vi "AlliGator Image Profile Menu Check Marks.vi"(8 "Error In":errorcluster, 11 "Menu in":refnum<k9>) -> (0 "Error Out":errorcluster)   [LabVIEW 2021, in "AlliGator Image Profile Window.lvlib"]
doc: "Handles checked items in Profile Window menu."
uses:
  AlliGator Image Profile Window.lvlib
  Globals, Variables, Constants/AlliGator Variables List.ctl
  Image/Box Profile Type.ctl
  AlliGator Image Profile Intensity Type.ctl
  AlliGator Image Profile Average Intensity Type.ctl
  Variant/Variant to Data/Variant to Boolean.vi
  Globals, Variables, Constants/AlliGator Globals, Variables & Constants.lvlib
  Variant/Variant to Data/Variant to Data.lvlib
  Image/Image.lvlib
panel:
  # "see the AlliGator License on the block diagram (Ctrl+E or Window:Show Block Diagram)"
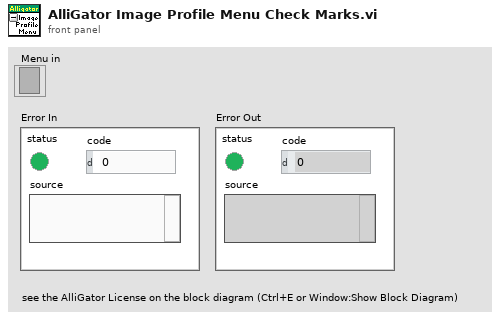
[diagram p1: front panel]
types:
  T1 = typedef "AlliGator Image Profile Window.lvlib/AlliGator Image Profile Average Intensity Type.ctl" = enum16{"Integrated Intensity", "Average Intensity", "Intensity-weighted Average Intensity"}
  T2 = typedef "AlliGator Image Profile Window.lvlib/AlliGator Image Profile Intensity Type.ctl" = enum16{"Raw Data", "Displayed Image", "Background-subtracted"}
  T3 = typedef "Image.lvlib/Box Profile Type.ctl" = enum16{"Full Width", "Half Width"}
  T4 = typedef "AlliGator Globals, Variables & Constants.lvlib/AlliGator Variables List.ctl" = enum16{"---- GUI ----", "GUI:Initialization Status", "GUI:State Indicators Refnum", "GUI:Original AlliGator Menu Items", "GUI:Current Action Loop State", "GUI:Script in progress", "GUI:Playback", "GUI:Loop Playback", "GUI:Search ROI Used", "GUI:Search ROI", "Decay Graph Max Legend Size", "Intensity Graph Max Legend Size", "Decay Statistics Graph Max Legend Size", "Phasor Graph Max Legend Size", "Phasor Ratio Graph Max Legend Size", "Lifetime Graph Max Legend Size", "---- Files ----", "Files:Export Dataset Frames as Individual Files", "Files:Show Batch Export Help Balloons", "Files:Frames in Dataset", "Files:ptu File Frame Start Indices", "Files:Current Frame in Dataset", "Files:Current Frame Timestamp", "Files:Dataset Loaded", "Files:Dataset Metadata", "Files:Dataset Channel", "Files:Dataset Data Description", "Files:Background Dataset Metadata", "Files:Background Dataset Channel", "Files:Background Dataset Data Description", "Files:Background File Subtraction", "Files:Background File Path", "Files:Background File Pile-up Correction", "Files:Background File Pixel Well Capacity", "Files:Background File Scaling Factor", "Files:Current Dataset Load Settings", "Files:Dataset Path", "Files:ICCD-specific Information", "Files:Macrotime Gate Separation", "------ Python Plugins ------", "Python Plugins:Information", "Python Plugins:Python Session", "Python Plugins:Valid Python Session?", "---- Source Image ----", "Source Image:ROIs", "Source Image:Current ROI", "Source Image:ROI Event Refnum", "X_Source Image Display Range", "X_Source Image Palette Information", "X_Type of Displayed Image", "X_Time Gate Slider", "Source Image:Palette List", "Source Image:Scale", "Source Image:ROI Overlay Color", "Source Image:Overlay to Erase", "Source Image:Is Displayed Image Accumulated", "Source Image:White Light Image Modified", "Source Image:Mask Image Modified", "---- Image Profile Window ----", "Image Profile:Window Event Refnum", "Image Profile:IntensityType", "Image Profile:Intensity Average Type", "Image Profile:Intensity-weighted SDV", "Image Profile:Box Profile Type", "Image Profile:Window Open", "Image Profile:Plotted Fit Parameter", "------ Phasor Graph -------", "Phasor Graph:Show Line", "---- Phasor Plot ---", "Phasor Plot:Parameters Changed", "Phasor Plot:FLI Dataset Modified since last Calculation", "Phasor Harmonics Data", "Selected Phasor Harmonics", "Phasor Harmonic Manager Event Refnum", "Phasor Plot:ROIs", "Phasor Plot:Current ROI", "Phasor Plot:ROI Event Refnum", "Phasor Plot:Image Reference Points", "Phasor Plot:Computed", "Phasor Plot:Palette Information", "Phasor Plot:Palette List", "Phasor Plot:Phasor Ratio Palette Information", "Phasor Plot:Phasor Ratio Palette List", "Phasor Plot:Image Scale", "Phasor Plot:Image Overlay to Erase", "Phasor Plot:Image Elements to Update", "Phasor Plot:Current Calculation Parameters", "Phasor Plot:Current Calibration Options", "Phasor Plot:Reset Cumulated Phasor Plot", "Phasor Plot:Reference 1", "Phasor Plot:Lifetime Reference 1", "Phasor Plot:Reference 1 Frequency", "Phasor Plot:Reference 2", "Phasor Plot:Lifetime Reference 2", "Phasor Plot:Reference 2 Frequency", "---- Decay Analysis ----", "Number of Selected Decays to Fit", "LS Fit Results", "LAR Fit Results", "BS Fit Results", "Last Decay Max - Min", "Best Fit Parameters", "Best Fit Parameter Names", "Actual Size X", "Actual Size Y", "Binning X", "Binning Y", "Actual # Gates", "Dataset Number", "Gates to...", "Gates Skipped", "Gates to keep", "Gate Step", "Gate Separation", "Reversed Gates", "Pile-up Correction", "Pixel Well Capacity", "Background Subtracted", "Background Subtraction Method", "Background Definition Range", "Background File (deprecated)", "Number of Dataset Accumulated", "Array of Accumulated Dataset Paths", "Do Averaged Datasets", "Destination File Path", "Process Plot Target", "Use 1/D as Phasor Frequency", "---- Decay Fit Parameter Map -----", "Decay Fit Parameter Map:Palette Information", "Decay Fit Parameter Map:Palette List", "---- Parameter Map ----", "Parameter Map:Palette Information", "Parameter Map:Palette List", "------- Local Decay Window ---------", "Local Decay Graph Window:Event Refnum", "Local Decay Graph Window:Use normalized IRF for convolution", "----- Miscellaneous ----", "Misc:Skippable Dialog Windows Status"}
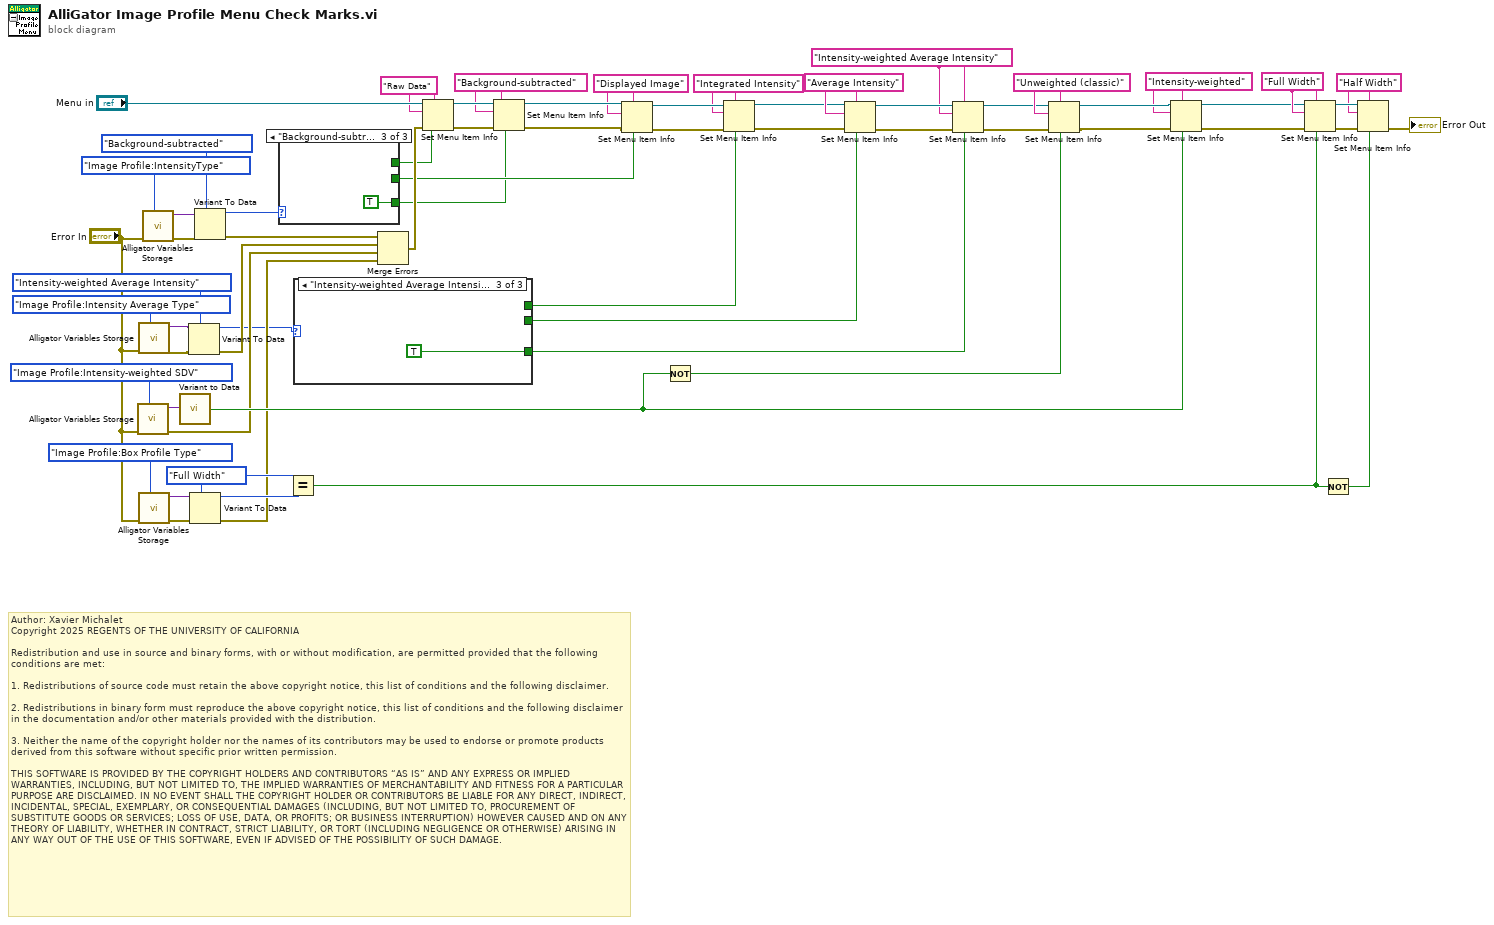
[diagram p0: block diagram]
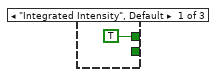
[diagram p2: hidden frame]
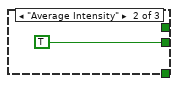
[diagram p3: hidden frame]
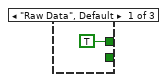
[diagram p4: hidden frame]
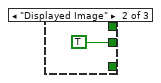
[diagram p5: hidden frame]
diagram:
  w2 = "Integrated Intensity" ("ItemTag")
  w9 = "Intensity-weighted Average Intensity" ("ItemTag")
  w10 = "Average Intensity" ("ItemTag")
  w39 = "Half Width" ("item tag")
  w37 = "Full Width" ("item tag")
  w41 = Box_Profile_Type."Full Width"
  w46 = "Intensity-weighted" ("ItemTag")
  w51 = "Unweighted (classic)" ("ItemTag")
  w54 = "Displayed Image" ("ItemTag")
  w58 = "Background-subtracted" ("ItemTag")
  w60 = "Raw Data" ("ItemTag")
  # "Author: Xavier Michalet\nCopyright 2025 REGENTS OF THE UNIVERSITY OF CALIFORNIA\n\nRedistribution and use in source and binary forms, with or without modification, are permitted provided that the following conditions are met:\n\n1. Redistributions of source code must retain the above copyright notice, this list of conditions and the following disclaimer.\n\n2. Redistributions in binary form must reproduce the above copyright notice, this list of conditions and the following disclaimer in the documentation and/or other materials provided with the distribution.\n\n3. Neither the name of the copyright holder nor the names of its contributors may be used to endorse or promote products derived from this software without specific prior written permission.\n\nTHIS SOFTWARE IS PROVIDED BY THE COPYRIGHT HOLDERS AND CONTRIBUTORS “AS IS” AND ANY EXPRESS OR IMPLIED WARRANTIES, INCLUDING, BUT NOT LIMITED TO, THE IMPLIED WARRANTIES OF MERCHANTABILITY AND FITNESS FOR A PARTICULAR PURPOSE ARE DISCLAIMED. IN NO EVENT SHALL THE COPYRIGHT HOLDER OR CONTRIBUTORS BE LIABLE FOR ANY DIRECT, INDIRECT, INCIDENTAL, SPECIAL, EXEMPLARY, OR CONSEQUENTIAL DAMAGES (INCLUDING, BUT NOT LIMITED TO, PROCUREMENT OF SUBSTITUTE GOODS OR SERVICES; LOSS OF USE, DATA, OR PROFITS; OR BUSINESS INTERRUPTION) HOWEVER CAUSED AND ON ANY THEORY OF LIABILITY, WHETHER IN CONTRACT, STRICT LIABILITY, OR TORT (INCLUDING NEGLIGENCE OR OTHERWISE) ARISING IN ANY WAY OUT OF THE USE OF THIS SOFTWARE, EVEN IF ADVISED OF THE POSSIBILITY OF SUCH DAMAGE."
  n1 = call "Alligator Variables Storage.vi"("AlliGator Variable"=AlliGator_Variables_List."Image Profile:Intensity-weighted SDV" ("Alligator Variable"), "Error In"="Error In") -> ("Error Out"=w31:errorcluster, "Data out"=w52:variant)  [unwired: 7 in, 1 out]
  n2 = call "Alligator Variables Storage.vi"("AlliGator Variable"=AlliGator_Variables_List."Image Profile:Intensity Average Type" ("Alligator Variable"), "Error In"="Error In") -> ("Error Out"=w19:errorcluster, "Data out"=w18:variant)  [unwired: 7 in, 1 out]
  n3 = call "Alligator Variables Storage.vi"("AlliGator Variable"=AlliGator_Variables_List."Image Profile:Box Profile Type" ("Alligator Variable"), "Error In"="Error In") -> ("Error Out"=w43:errorcluster, "Data out"=w44:variant)  [unwired: 7 in, 1 out]
  n4 = call "Alligator Variables Storage.vi"("AlliGator Variable"=AlliGator_Variables_List."Image Profile:IntensityType" ("Alligator Variable"), "Error In"="Error In") -> ("Error Out"=w26:errorcluster, "Data out"=w27:variant)  [unwired: 7 in, 1 out]
  n5 = call-poly "Variant to Data.vi"("Variant"=w52) -> ("Value"=w48:bool)  [unwired: 8 in]
  n6 = Variant To Data(error in=w19, type=AlliGator_Image_Profile_Average_Intensity_Type."Intensity-weighted Average Intensity" ("Image Profile Average Intenisty Type"), Variant=w18) -> (data=w15:T1, error out=w17:errorcluster)
  n7 = Variant To Data(error in=w43, type=w41, Variant=w44) -> (data=w42:T3, error out=w30:errorcluster)
  n8 = Variant To Data(error in=w26, type=AlliGator_Image_Profile_Intensity_Type."Background-subtracted" ("Image Profile Intensity Type"), Variant=w27) -> (data=w23:T2, error out=w25:errorcluster)
  n9 = case shown="\"Background-subtracted\"" w23 {
    tunnel: [TRUE _ _] -> w22
    tunnel: [_ TRUE _] -> w21
    tunnel: [_ _ TRUE] -> w20
    frame "Raw Data", Default {
    }
    frame "Displayed Image" {
    }
    frame "Background-subtracted" {
    }
  }
  n10 = Equal?(x=w41, y=w42) -> (x = y?=w34:bool)
  n11 = case shown="\"Intensity-weighted Average Intensity\"" w15 {
    tunnel: [_ TRUE _] -> w8
    tunnel: [_ _ TRUE] -> w7
    tunnel: [TRUE _ _] -> w1
    frame "Integrated Intensity", Default {
    }
    frame "Average Intensity" {
    }
    frame "Intensity-weighted Average Intensity" {
    }
  }
  n12 = Merge Errors(w25, w17, w31, w30) -> (w32:errorcluster)
  n13 = Set Menu Item Info(6:w22, 7:w60, 8:w32, 10:w60, 11:"Menu in") -> (0:w57:errorcluster, 3:w59:refnum<k9>)  [unwired: 2 in]
  n14 = Set Menu Item Info(6:w20, 7:w58, 8:w57, 10:w58, 11:w59) -> (0:w55:errorcluster, 3:w56:refnum<k9>)  [unwired: 2 in]
  n15 = Set Menu Item Info(6:w21, 7:w54, 8:w55, 10:w54, 11:w56) -> (0:w6:errorcluster, 3:w4:refnum<k9>)  [unwired: 2 in]
  n16 = Not(x=w48) -> (.not. x?=w47:bool)
  n17 = Set Menu Item Info(6:w1, 7:w2, 8:w6, 10:w2, 11:w4) -> (0:w5:errorcluster, 3:w3:refnum<k9>)  [unwired: 2 in]
  n18 = Set Menu Item Info(6:w8, 7:w10, 8:w5, 10:w10, 11:w3) -> (0:w14:errorcluster, 3:w12:refnum<k9>)  [unwired: 2 in]
  n19 = Set Menu Item Info(6:w7, 7:w9, 8:w14, 10:w9, 11:w12) -> (0:w13:errorcluster, 3:w11:refnum<k9>)  [unwired: 2 in]
  n20 = Set Menu Item Info(6:w47, 7:w51, 8:w13, 10:w51, 11:w11) -> (0:w49:errorcluster, 3:w50:refnum<k9>)  [unwired: 2 in]
  n21 = Set Menu Item Info(6:w48, 7:w46, 8:w49, 10:w46, 11:w50) -> (0:w35:errorcluster, 3:w36:refnum<k9>)  [unwired: 2 in]
  n22 = Set Menu Item Info(6:w34, 7:w37, 8:w35, 10:w37, 11:w36) -> (0:w38:errorcluster, 3:w40:refnum<k9>)  [unwired: 2 in]
  n23 = Not(x=w34) -> (.not. x?=w33:bool)
  n24 = Set Menu Item Info(6:w33, 7:w39, 8:w38, 10:w39, 11:w40) -> (0:→"Error Out":errorcluster)  [unwired: 2 in, 1 out]
